vi "test Error Code.vi"(8 "error in (no error)":errorcluster, 11 "TestCase in":refnum<class "Parameter Setting.lvclass">) -> (0 "error out":errorcluster, 3 "TestCase out":refnum<class "Parameter Setting.lvclass">)   [LabVIEW 2017, in "Static Errors Tests.lvlib" / "Parameter Setting.lvclass"]
uses:
  Parameter Setting.lvclass
  Parameter Setting.lvclass/Parameter Setting.ctl
  <vilib>/addons/_JKI Toolkits/VI Tester/TestCase.llb/TestCase.lvclass
  Source/Static Errors.lvlib
  C:/Program Files (x86)/National Instruments/LabVIEW 2017/vi.lib/addons/_JKI Toolkits/VI Tester/TestCase.llb/TestCase.lvclass
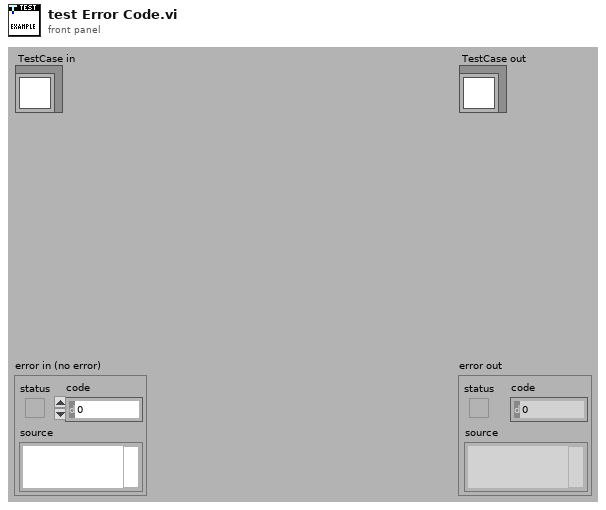
[diagram p1: front panel]
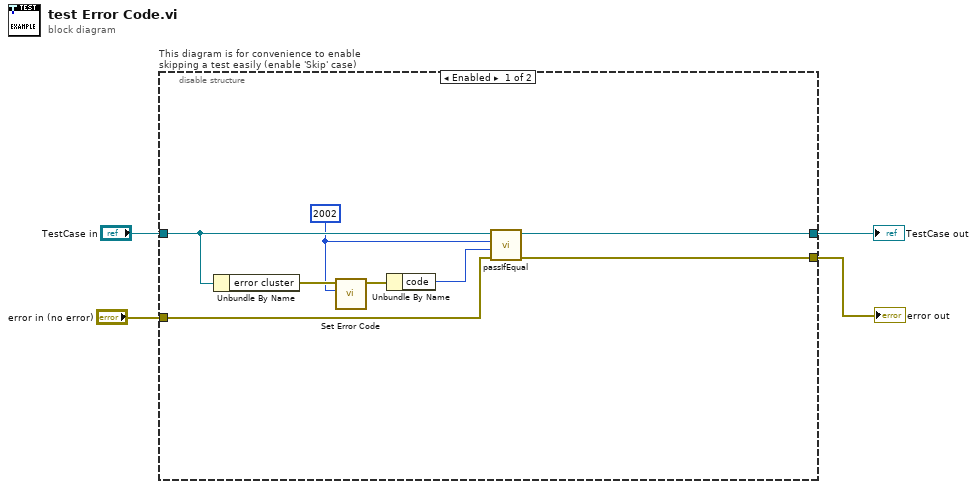
[diagram p0: block diagram]
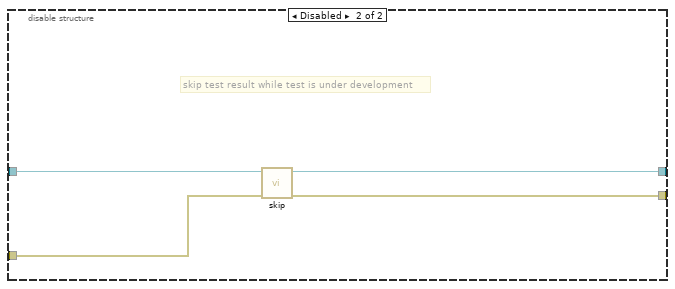
[diagram p2: hidden frame]
diagram:
  n1 = disable-structure "This diagram is for convenience to enable skipping a test easily (enable 'Skip' case)" shown="Enabled" {
    disable-tunnel: "TestCase in" -> [w10 w16]
    disable-tunnel: [w12 w14] -> w2
    disable-tunnel: [w11 w15] -> w1
    disable-tunnel: "error in (no error)" -> [w5 w13]
    frame Enabled {
      w6 = 2002 ("code")
      n2 = Unbundle By Name(w10) -> ("error cluster"=w8:errorcluster)
      n3 = call "Set Error Code.vi"("code"=w6, "error in"=w8) -> ("error out"=w7:errorcluster)  [unwired: 8 in, 1 out]
      n4 = Unbundle By Name(w7) -> ("code"=w9:i32)
      n5 = call-dynamic "passIfEqual.vi"("error in (no error)"=w5, "y"=w9, "x"=w6, "TestCase in"=w10) -> ("error out"=w11:errorcluster, "TestCase out"=w12:refnum<class "Parameter Setting.lvclass">)  [unwired: 6 in]
    }
    frame Disabled {
      # "skip test result while test is under development"
      n6 = call <vilib>:"skip.vi"("error in (no error)"=w13, "TestCase in"=w16) -> ("error out"=w15:errorcluster, "TestCase out"=w14:refnum<class "Parameter Setting.lvclass">)  [unwired: 8 in]
    }
  }
  "error out" <- w1
  "TestCase out" <- w2
